vi "Update Status Counter.vi"(10 "Result":T1={"Name"="", "Message"="", "Description"="", "Status"=enum."Passed", "Result Type"=enum."Case", "Execution Time"=0.0}, 11 "Result Model in":refnum<class "Result Model.lvclass">) -> (3 "Result Model out":refnum<class "Result Model.lvclass">)   [LabVIEW 2020, in "Result Model.lvclass"]
uses:
  Result Model.lvclass
  Result/Result.ctl
  Result/Status.ctl
  Result/Type.ctl
  Result Model.lvclass/Result Model.ctl
  <vilib>/Utility/miscctls.llb/LVMapReplaceAction.ctl
  Utilities/LUnit Utilities.lvlib
  Result/Result.lvlib
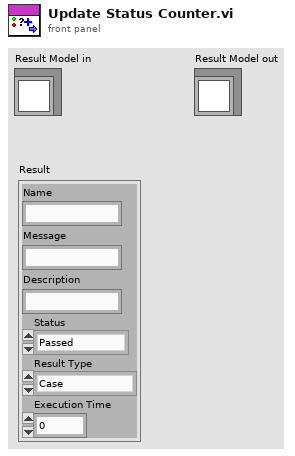
[diagram p1: front panel]
types:
  T1 = typedef "Result.lvlib/Result.ctl" = cluster{"Name":string, "Message":string, "Description":string, "Status":T2, "Result Type":T3, "Execution Time":dbl}
  T2 = typedef "Result.lvlib/Status.ctl" = enum16{"", "Passed", "Failed", "Error", "Skipped", "Setup Error", "Broken", "Teardown Error"}
  T3 = typedef "Result.lvlib/Type.ctl" = enum16{"Method", "Case", "Suite", "Pass", "Fail", "Skip", "Pass if", "Fail if", "Pass if Error", "Fail if Error", "Pass if Equal", "Fail if Equal"}
  T4 = typedef "LVMapReplaceAction.ctl" = enum32{"Modify Entry only if found", "Add or Modify Entry", "Delete Entry"}
  T5 = map{cluster{"Test Case":string, "Status":T2}, i32}
  T6 = cluster{"Test Case Class Name":string, "Status":T2}
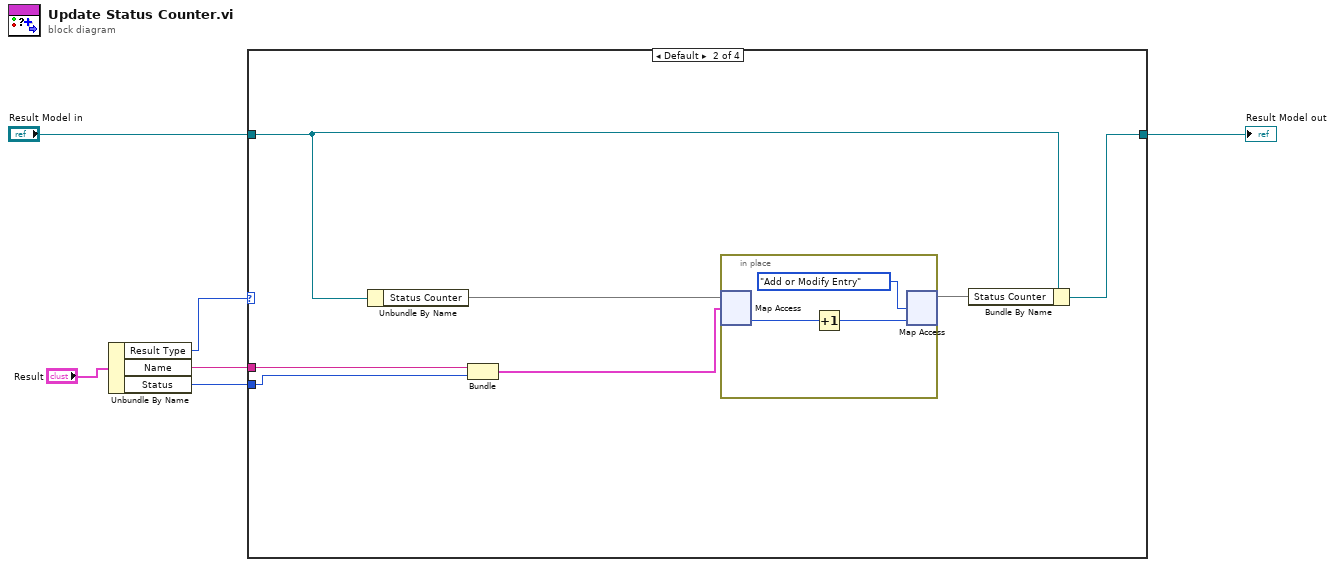
[diagram p0: block diagram]
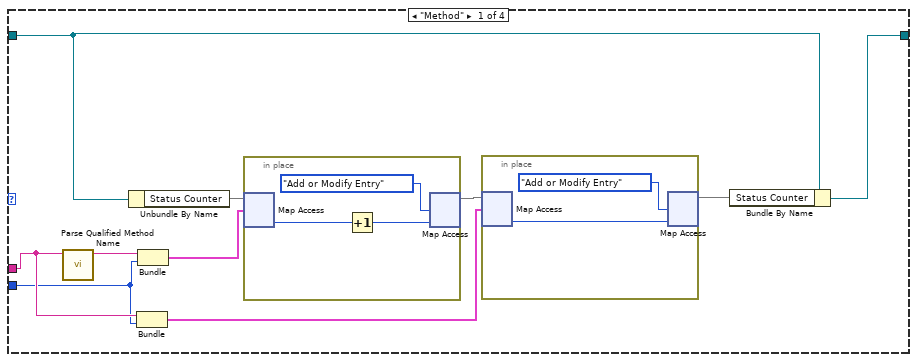
[diagram p2: hidden frame]
diagram:
  n1 = Unbundle By Name("Result") -> ("Result Type"=w1:T3, "Name"=w4:string, "Status"=w5:T2)
  n2 = case shown="Default" w1 {
    tunnel: w5 -> [w8 w23 _ _]
    tunnel: w4 -> [w9 w24 _ _]
    tunnel: "Result Model in" -> [w13 w27 w32 w33]
    tunnel: [w12 w26 w32 w33] -> w2
    frame "Method" {
      n3 = call "Parse Qualified Method Name.vi"("Case"=w9) -> ("Test Case Class Name"=w14:string)  [unwired: 9 in, 1 out]
      n4 = Unbundle By Name(w13) -> ("Status Counter"=w16:T5)
      n5 = Bundle("Name"=w9, "Status"=w8) -> (w7:cluster{"Name":string, "Status":T2})  [unwired: 1 in]
      n6 = Bundle("Test Case Class Name"=w14, "Status"=w8) -> (w10:T6)  [unwired: 1 in]
      n7 = in-place {
        n8 = in-place-map #1(w16, w10) -> (w21:i32)  [unwired: 1 in, 1 out]
        n9 = Increment(x=w21) -> (x+1=w20:i32)
        n10 = in-place-map #1(w20, LVMapReplaceAction."Add or Modify Entry" ("action")) -> (w15:T5)  [unwired: 2 out]
      }
      n11 = in-place {
        n12 = in-place-map #2(w15, w7) -> (w18:i32)  [unwired: 1 in, 1 out]
        n13 = in-place-map #2(w18, LVMapReplaceAction."Add or Modify Entry" ("action")) -> (w11:T5)  [unwired: 2 out]
      }
      n14 = Bundle By Name(cluster=w13, "Status Counter"=w11) -> (w12:refnum<class "Result Model.lvclass">)
    }
    frame Default {
      n15 = Unbundle By Name(w27) -> ("Status Counter"=w28:T5)
      n16 = Bundle("Name"=w24, "Status"=w23) -> (w22:cluster{"Name":string, "Status":T2})  [unwired: 1 in]
      n17 = in-place {
        n18 = in-place-map #3(w28, w22) -> (w31:i32)  [unwired: 1 in, 1 out]
        n19 = Increment(x=w31) -> (x+1=w29:i32)
        n20 = in-place-map #3(w29, LVMapReplaceAction."Add or Modify Entry" ("action")) -> (w25:T5)  [unwired: 2 out]
      }
      n21 = Bundle By Name(cluster=w27, "Status Counter"=w25) -> (w26:refnum<class "Result Model.lvclass">)
    }
    frame "Case" {
    }
    frame "Suite" {
    }
  }
  "Result Model out" <- w2
